vi "CMC_Numeric_Controls_and_Indicators.vi"() -> ()   [LabVIEW 2013]
panel:
  out "Indicator":dbl
  in  "Control 2":dbl min=0.0 max=100.0 step=1.0
  in  "Control 1":dbl min=0.0 max=100.0 step=1.0
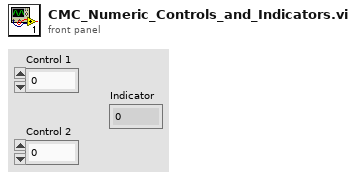
[diagram p1: front panel]
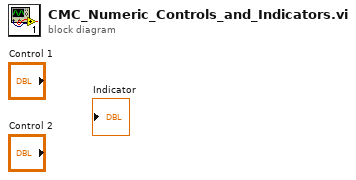
[diagram p0: block diagram]
diagram:
